vi "Connect.vi"(8 "error in (no error)":errorcluster, 11 "DG645 in":refnum<class "DG645.lvclass">) -> (0 "error out":errorcluster, 3 "DG645 out":refnum<class "DG645.lvclass">)   [LabVIEW 2018, in "DG645.lvlib" / "DG645.lvclass"]
uses:
  DG645.lvclass
  DG645.lvclass/DG645.ctl
  <instrlib>/Stanford Research DG645/Stanford Research DG645.lvlib
  PPLs/Digital Delay Generator/Parent/Digital Delay Generator.lvlibp/Digital Delay Generator.lvclass
  C:/AME Test Engineering/LabVIEW/PPLs/Digital Delay Generator/Parent/Digital Delay Generator.lvlibp/Digital Delay Generator.lvclass
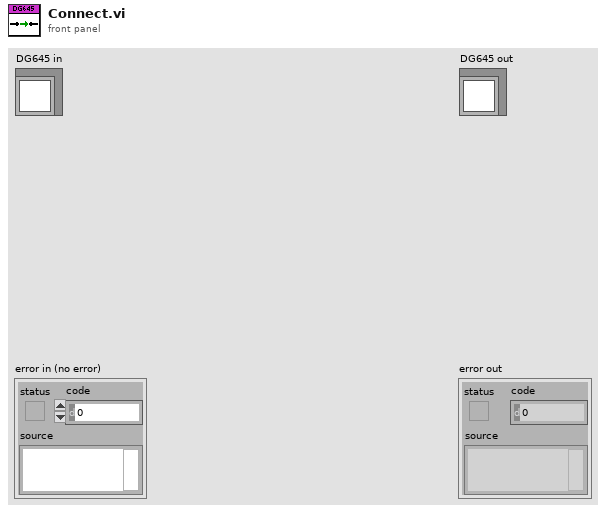
[diagram p1: front panel]
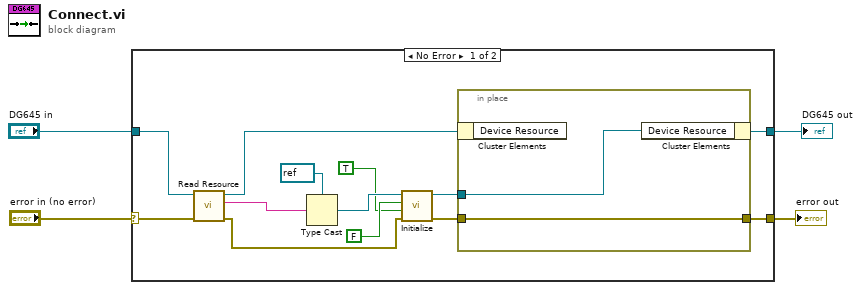
[diagram p0: block diagram]
diagram:
  n1 = case shown="No Error" "error in (no error)" {
    selector: "error in (no error)" -> [w8 w20]
    tunnel: "DG645 in" -> [w10 w21]
    tunnel: [w12 w21] -> w2
    tunnel: [w11 w20] -> w1
    frame No Error {
      n2 = call "Read Resource.vi"("error in (no error)"=w8, "Digital Delay Generator in"=w10) -> ("error out"=w6:errorcluster, "Resource"=w7:string, "Digital Delay Generator out"=w9:refnum<class "DG645.lvclass">)  [unwired: 7 in]
      n3 = Type Cast(type=refnum<visa-resource-name> refnum ("VISA resource name"), x=w7) -> (*(type *) &x=w16:refnum<visa-resource-name>)
      n4 = call <instrlib>:"Initialize.vi"("error in (no error)"=w6, "Reset (True)"=TRUE, "ID Query (True)"=FALSE, "VISA resource name"=w16) -> ("error out"=w14:errorcluster, "VISA resource name out"=w13:refnum<visa-resource-name>)  [unwired: 6 in]
      n5 = in-place {
        in-place-border: w14 -> [w18]
        in-place-border: w13 -> [w19]
        in-place-border: [w18] -> w11
        n6 = in-place-cluster #1(w9) -> ()  [unwired: 1 out]
        n7 = in-place-cluster #1("Device Resource"=w19) -> (w12:refnum<class "DG645.lvclass">)
      }
    }
    frame Error {
    }
  }
  "error out" <- w1
  "DG645 out" <- w2
